vi "WSVCAP SHL FPGA LL SPI Debug Global.vi"() -> ()   [LabVIEW 2012]
panel:
  out "Sim Write Memory":u16[](array[numeric]) format="%08x"
  in  "SPI CH (1-16)":i32
  in  "SPI_DATO":bool
  in  "SPI_DAA":bool
  in  "SPI_EN":bool
  in  "SPI_CLK":bool
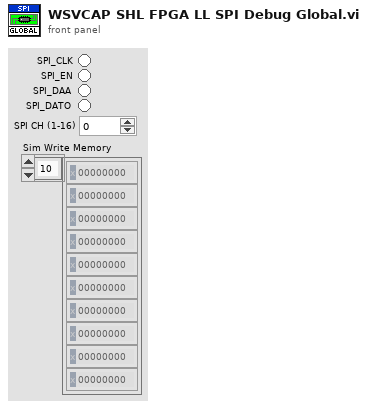
[diagram p1: front panel]
diagram:
